vi "onAssertionSlippage.vi"(7 "AssertTrue in":refnum<class "AssertTrue.lvclass">, 11 "Leaf.Assertion":refnum<class "Leaf.Assertion.lvclass">) -> (0 "error out":errorcluster, 3 "Leaf.Assertion":refnum<class "Leaf.Assertion.lvclass">)   [LabVIEW 2021, in "Bananas.lvlib" / "AssertTrue.lvclass"]
uses:
  AssertTrue.lvclass
  Leaf.Assertion/Leaf.Assertion.lvclass
  C:/Repositories/LVOS/Bananas/lv-src/Bananas/Leaf/Leaf.lvclass
  AssertTrue.lvclass/AssertTrue.ctl
  Leaf/Leaf.lvclass
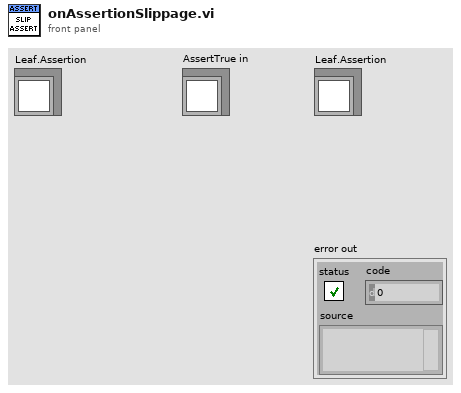
[diagram p1: front panel]
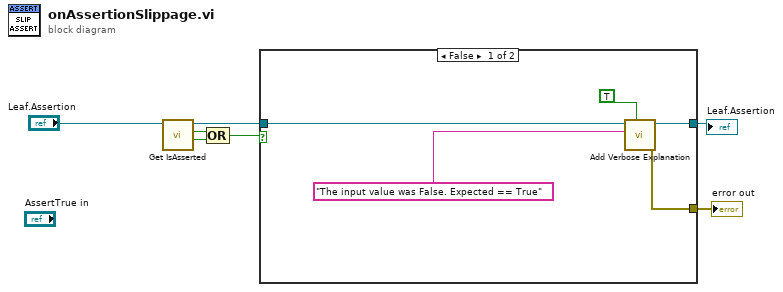
[diagram p0: block diagram]
diagram:
  n1 = call "Get IsAsserted.vi"("Leaf.Assertion"="Leaf.Assertion") -> ("Skipped"=w4:bool, "Asserted"=w5:bool, "Leaf.Assertion"=w2:refnum<class "Leaf.Assertion.lvclass">)  [unwired: 8 in]
  n2 = Compound Arithmetic op=OR(w5, w4) -> (w1:bool)
  n3 = case shown="False" w1 {
    tunnel: [w9 w13] -> w7
    tunnel: [w8 _] -> w6
    tunnel: w2 -> [w12 w13]
    frame False {
      n4 = call "Add Verbose Explanation.vi"("overwrite"=TRUE ("overwrite?"), "Verbose Explanation"="The input value was False. Expected == True", "Leaf in"=w12) -> ("error out"=w8:errorcluster, "Leaf out"=w9:refnum<class "Leaf.Assertion.lvclass">)  [unwired: 7 in]
    }
    frame True {
      # "There was an upstream error or the assertion = TRUE"
    }
  }
  "error out" <- w6
  "Leaf.Assertion" <- w7
